vi "pco.camera_LightSheet_Example.vi"() -> ()   [LabVIEW 2020]
uses:
  Camera.lvclass
  SpecialCommandsEdge.lvlib
panel:
  out "colormap(U8)":u32[](array[numeric])
  out "Image(U16)":u16[][](graph)
  in  "Zoom [%]":i32(c297)=26
  out "Image":picture
  in  "dwExposureLines":u32=100
  in  "wTimeBase":u16(ring)=1 items=["ns", "us", "ms"]
  in  "dwLineTime":u32=50
  out "rawImage":u16[][](array[numeric])
  in  "data_format":T1(ring)=enum."Mono16"
  in  "Image Index":u32 max=9
  out "Recorded Images":u32
  in  "Quit":bool
  in  "roiY1":u64=2 min=2 max=2160 step=1
  in  "roiX1":u64=2 min=2 max=2560 step=1
  in  "roiY0":u64=1 min=1 max=2159 step=1
  in  "roiX0":u64=1 min=1 max=2559 step=1
  out "Image Height":u64
  out "Image Width":u64
  in  "dwImgCount":u32=10 caption="Required Number of Images" max=4023
  out "Error":errorcluster {"code" format="%x"}
  # "This example is similar to the simple example, but uses get/set line timeing for controlling the exposure.\nExposureTime = LineTime * ExposureLines\nBeside of the line timing part, a simple recording of an image sequence and the image access afterwards is done.\nIt is a good starting point for writing own applications, especially  for light sheet application development.\nBut it will not be fail save, i.e. doesnt react on errors, just handles them forward to the end\n\nUsage:\nSelect your required image count and the required line tiime + number of exposure lines before you start the program.\nOnce started, the camera class will be initialized and images will be recorded automatically.\nWhen acquisition has finished you can address the images and set a certain roi \nTo finish the program click on quit application, this will force fan exit of the camera class"
  # "pco.labview"
  # "Camera Setup"
  # "Recording Control"
  # "Parameters for image readout"
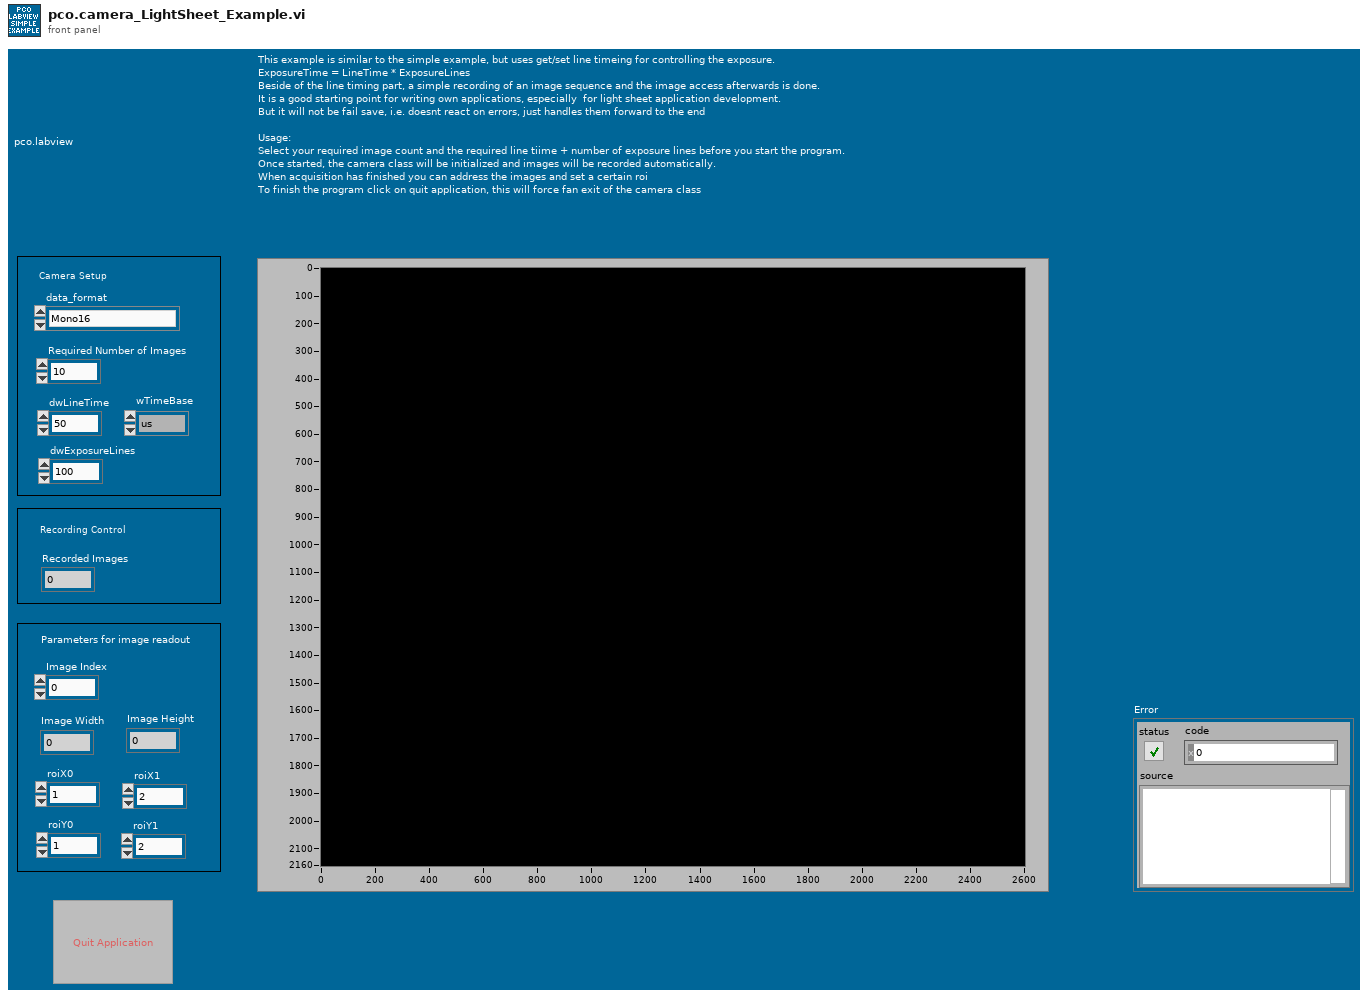
[diagram p1: front panel]
types:
  T1 = enum16{"Undefined", "Mono8", "Mono16", "BGRA8", "RGBA8", "BGRA16", "RGBA16", "CompressedMono8"}
  T2 = enum8{"Enabled", "Disabled", "Disabled and Grayed Out"}
  T3 = enum16{"sequence", "sequence non blocking", "ring buffer", "fifo", "sequence_dpcore", "sequence_non_blocking_dpcore", "ring_buffer_dpcore", "fifo_dpcore", "tif", "multitif", "pcoraw", "b16", "dicom", "multidicom"}
  T4 = typedef "Camera.lvclass/binning.ctl" = cluster{"vert":u16, "horz":u16}
  T5 = cluster{"exposure_time_s":dbl, "delay_time_s":dbl, "roi":cluster{"x0":u64, "y0":u64, "x1":u64, "y1":u64}, "timestamp_mode":u16, "pixelrate":u32, "trigger_mode":u16, "acquire_mode":u16, "metadata_mode":u16, "noisefilter_mode":u16, "binning":T4}
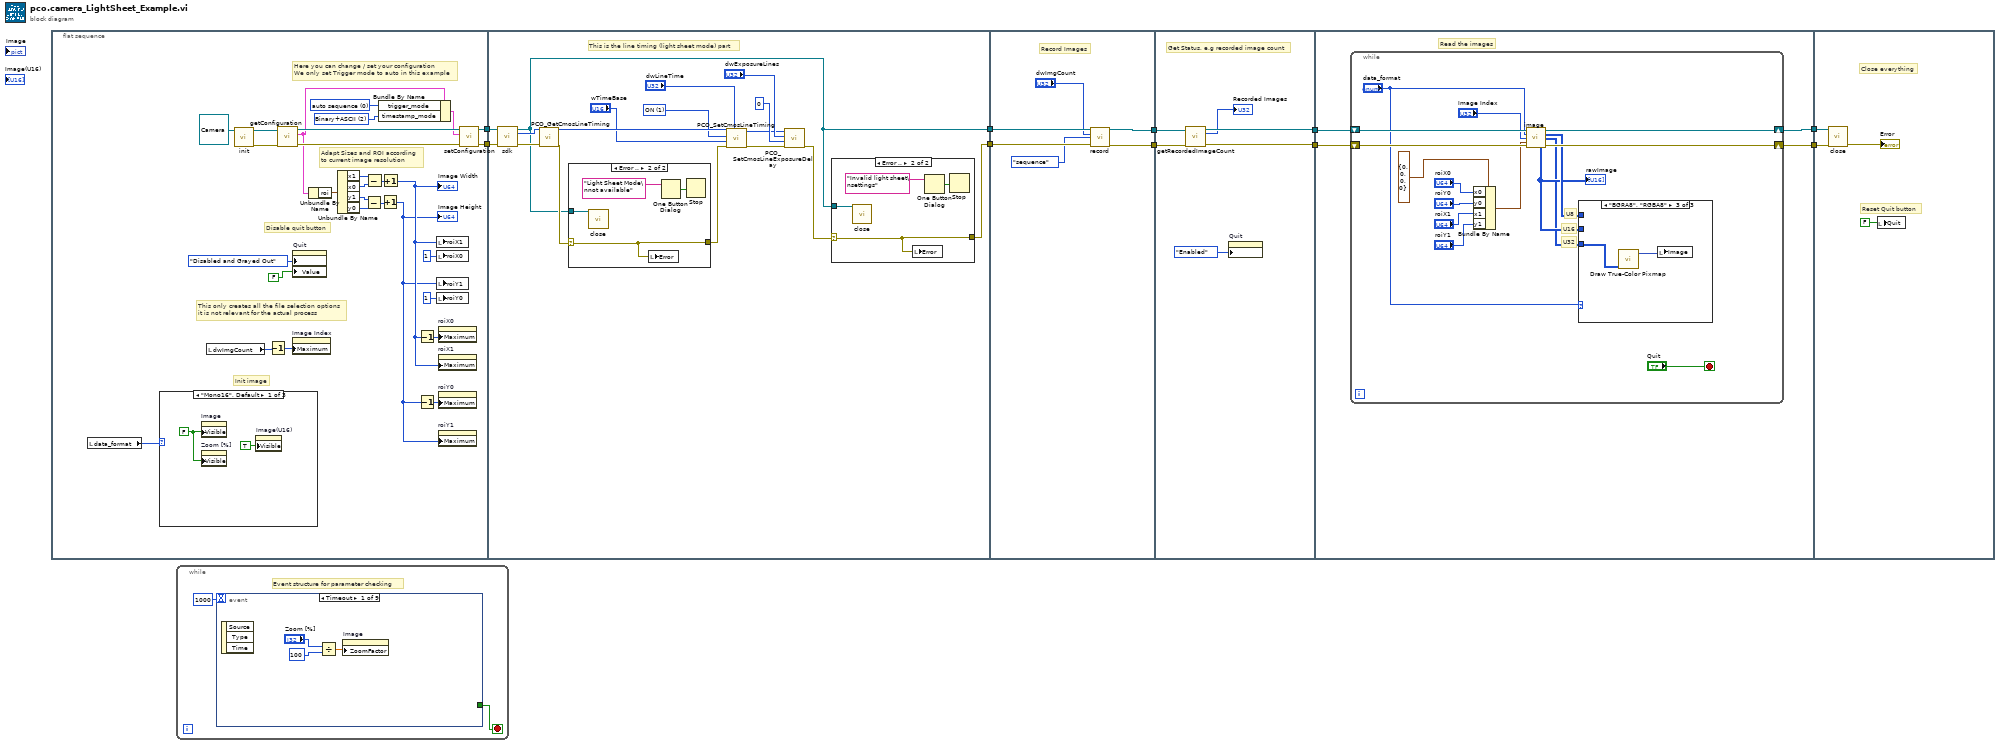
[diagram p0: block diagram]
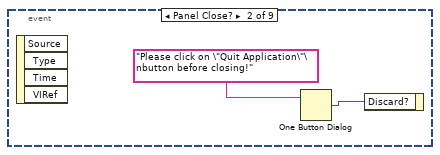
[diagram p2: hidden frame]
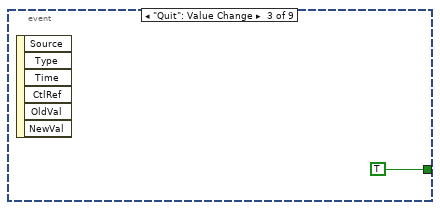
[diagram p3: hidden frame]
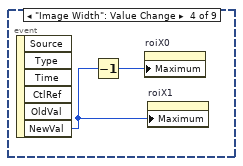
[diagram p4: hidden frame]
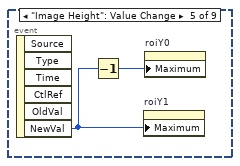
[diagram p5: hidden frame]
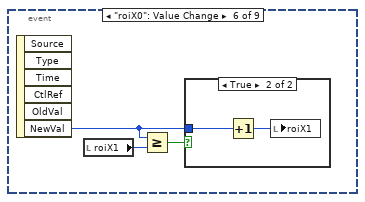
[diagram p6: hidden frame]
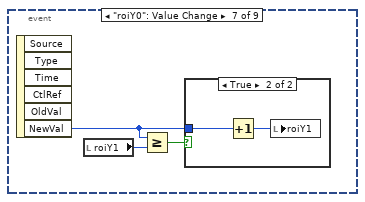
[diagram p8: hidden frame]
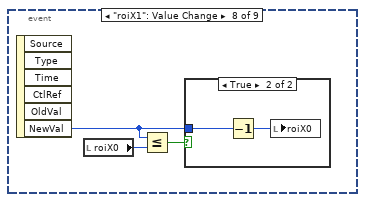
[diagram p10: hidden frame]
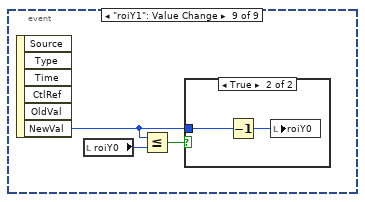
[diagram p12: hidden frame]
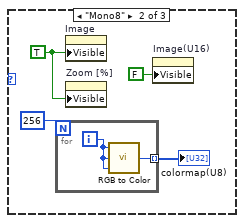
[diagram p14: hidden frame]
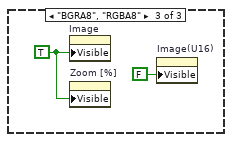
[diagram p15: hidden frame]
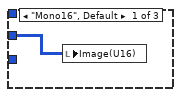
[diagram p18: hidden frame]
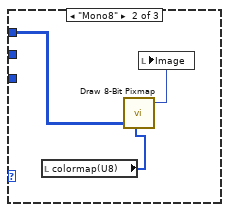
[diagram p19: hidden frame]
diagram:
  n1 = flat-sequence {
    tunnel: [w32] -> w4
    tunnel: [w31] -> w2
    tunnel: w4 -> [w62]
    tunnel: [w52] -> w3
    tunnel: w2 -> [w61]
    tunnel: [w50] -> w1
    tunnel: w3 -> [w82]
    tunnel: w1 -> [w81]
    tunnel: [w79] -> w10
    tunnel: [w78] -> w9
    tunnel: w10 -> [w88]
    tunnel: w9 -> [w87]
    tunnel: [w86] -> w8
    tunnel: [w85] -> w7
    tunnel: w8 -> [w91]
    tunnel: w7 -> [w92]
    tunnel: [w90] -> w6
    tunnel: [w89] -> w5
    tunnel: w6 -> [w116]
    tunnel: w5 -> [w115]
    frame #0 {
      w16 = u16 2 items=["OFF", "Binary", "Binary+ASCII", "ASCII"] ("TimestampMode")
      w36 = u16 0 items=["auto sequence"=0, "software trigger"=1, "external exposure start & software trigger"=2, "external exposure control"=3, "external synchronized"=4, "fast external exposure control"=5, "external CDS control"=6, "slow external exposure control"=7, "external synchronized HDSDI"=258] ("TriggerMode")
      # "Init image"
      # "This only creates all the file selection options\nit is not relevant for the actual process"
      # "Adapt Sizes and ROI according\nto current image resolution"
      # "Disable quit button"
      # "Here you can change / set your configuration\nWe only set Trigger mode to auto in this example"
      n2 = local read "data_format"() -> (w11:T1)
      n3 = case shown="\"Mono16\", Default" w11 {
        frame "Mono16", Default {
          w40 = FALSE ("Visible")
          n4 = property on="Image" class="Pict"("Visible"=w40) -> ()  [unwired: 2 in, 2 out]
          n5 = property on="Zoom [%]" class="Scroll (strict)"("Visible"=w40) -> ()  [unwired: 2 in, 2 out]
          n6 = property on="Image(U16)" class="IntGraph (strict)"("Visible"=TRUE) -> ()  [unwired: 2 in, 2 out]
        }
        frame "Mono8" {
          w44 = TRUE ("Visible")
          n7 = for {
            N: 256 -> [_]
            tunnel: [w46] -> w43 mode=indexing
            i -> [w47]
            n8 = call "RGB to Color.vi"("B"=w47, "G"=w47, "R"=w47) -> ("Color"=w46:u32)
          }
          "colormap(U8)" <- w43
          n9 = property on="Image" class="Pict"("Visible"=w44) -> ()  [unwired: 2 in, 2 out]
          n10 = property on="Zoom [%]" class="Scroll (strict)"("Visible"=w44) -> ()  [unwired: 2 in, 2 out]
          n11 = property on="Image(U16)" class="IntGraph (strict)"("Visible"=FALSE) -> ()  [unwired: 2 in, 2 out]
        }
        frame "BGRA8", "RGBA8" {
          w48 = TRUE ("Visible")
          n12 = property on="Image" class="Pict"("Visible"=w48) -> ()  [unwired: 2 in, 2 out]
          n13 = property on="Zoom [%]" class="Scroll (strict)"("Visible"=w48) -> ()  [unwired: 2 in, 2 out]
          n14 = property on="Image(U16)" class="IntGraph (strict)"("Visible"=FALSE) -> ()  [unwired: 2 in, 2 out]
        }
      }
      n15 = local read "dwImgCount"() -> (w12:u32)
      n16 = call-dynamic "init.vi"("Camera in"=refnum<class "Camera.lvclass"> refnum ("PCOCamera in")) -> ("Camera out"=w38:refnum<class "Camera.lvclass">, "error out"=w37:errorcluster)  [unwired: 8 in]
      n17 = Decrement(x=w12) -> (x-1=w13:u32)
      n18 = call-dynamic "getConfiguration.vi"("error in (no error)"=w37, "Camera in"=w38) -> ("error out"=w34:errorcluster, "configuration"=w26:T5, "Camera out"=w35:refnum<class "Camera.lvclass">)  [unwired: 7 in]
      n19 = property on="Image Index" class="DigNum (strict)"("Maximum"=w13) -> ()  [unwired: 2 in, 2 out]
      n20 = property on="Quit" class="Bool (strict)"("DisabledEnum"=T2."Disabled and Grayed Out" ("Disabled"), "Value"=FALSE ("Stop")) -> ()  [unwired: 2 in, 2 out]
      n21 = Unbundle By Name(w26) -> ("roi"=w25:cluster{"x0":u64, "y0":u64, "x1":u64, "y1":u64})
      n22 = Unbundle By Name(w25) -> ("x1"=w23:u64, "x0"=w24:u64, "y1"=w21:u64, "y0"=w22:u64)
      n23 = Subtract(x=w21, y=w22) -> (x-y=w19:u64)
      n24 = Subtract(x=w23, y=w24) -> (x-y=w20:u64)
      n25 = Bundle By Name(cluster=w26, "trigger_mode"=w36, "timestamp_mode"=w16) -> (w33:T5)
      n26 = Increment(x=w19) -> (x+1=w17:u64)
      "Image Height" <- w17
      n27 = Increment(x=w20) -> (x+1=w18:u64)
      "Image Width" <- w18
      n28 = Decrement(x=w18) -> (x-1=w28:u64)
      n29 = Decrement(x=w17) -> (x-1=w27:u64)
      n30 = local write "roiX1"(w18) -> ()
      n31 = local write "roiX0"(u64 1 ("roiY0")) -> ()
      n32 = local write "roiY1"(w17) -> ()
      n33 = local write "roiY0"(u64 1 ("roiY0")) -> ()
      n34 = property on="roiX0" class="DigNum (strict)"("Maximum"=w28) -> ()  [unwired: 2 in, 2 out]
      n35 = property on="roiX1" class="DigNum (strict)"("Maximum"=w18) -> ()  [unwired: 2 in, 2 out]
      n36 = property on="roiY0" class="DigNum (strict)"("Maximum"=w27) -> ()  [unwired: 2 in, 2 out]
      n37 = property on="roiY1" class="DigNum (strict)"("Maximum"=w17) -> ()  [unwired: 2 in, 2 out]
      n38 = call-dynamic "setConfiguration.vi"("error in (no error)"=w34, "configuration"=w33, "Camera in"=w35) -> ("error out"=w31:errorcluster, "Camera out"=w32:refnum<class "Camera.lvclass">)  [unwired: 7 in]
    }
    frame #1 {
      w58 = u16 1 items=["OFF", "ON"] ("wParameter")
      # "This is the line timing (light sheet mode) part"
      n39 = call-dynamic "sdk.vi"("Camera in"=w62, "error in (no error)"=w61) -> ("Camera out"=w52:refnum<class "Camera.lvclass">, "sdk"=w60:u64, "error out"=w66:errorcluster)  [unwired: 11 in]
      n40 = call "PCO_GetCmosLineTiming.vi"("ph"=w60, "error in (no error)"=w66) -> ("ph out"=w59:u64, "error out"=w65:errorcluster)  [unwired: 10 in, 6 out]
      n41 = case shown="Error .." w65 {
        selector: w65 -> [w72 w73]
        tunnel: [w72 w73] -> w64
        tunnel: w52 -> [_ w74]
        frame No Error {
        }
        frame Error {
          n42 = call-dynamic "close.vi"("Camera in"=w74) -> ()  [unwired: 10 in, 1 out]
          n43 = local write "Error"(w73) -> ()
          n44 = One Button Dialog(message="Light Sheet Mode\nnot available") -> (true=w75:bool)  [unwired: 1 in]
          n45 = Stop(stop? (T)=w75) -> ()
        }
      }
      n46 = call "PCO_SetCmosLineTiming.vi"("dwLineTime"="dwLineTime", "error in (no error)"=w64, "wTimeBase"="wTimeBase", "wParameter"=w58, "ph"=w59) -> ("error out"=w63:errorcluster, "ph out"=w53:u64)  [unwired: 4 in, 1 out]
      n47 = call "PCO_SetCmosLineExposureDelay.vi"("error in (no error)"=w63, "dwDelayLines"=u32 0, "dwExposureLines"="dwExposureLines", "ph"=w53) -> ("error out"=w51:errorcluster)  [unwired: 5 in, 2 out]
      n48 = case shown="Error .." w51 {
        selector: w51 -> [w67 w68]
        tunnel: [w67 w68] -> w50
        tunnel: w52 -> [_ w69]
        frame No Error {
        }
        frame Error {
          n49 = call-dynamic "close.vi"("Camera in"=w69) -> ()  [unwired: 10 in, 1 out]
          n50 = local write "Error"(w68) -> ()
          n51 = One Button Dialog(message="Invalid light sheet\nsettings") -> (true=w70:bool)  [unwired: 1 in]
          n52 = Stop(stop? (T)=w70) -> ()
        }
      }
    }
    frame #2 {
      # "Record Images"
      n53 = call-dynamic "record.vi"("Camera in"=w82, "num_images"="dwImgCount", "record_mode"=T3."sequence", "error in (no error)"=w81) -> ("Camera out"=w79:refnum<class "Camera.lvclass">, "error out"=w78:errorcluster)  [unwired: 10 in]
    }
    frame #3 {
      # "Get Status, e.g recorded image count"
      n54 = call-dynamic "getRecordedImageCount.vi"("Camera in"=w88, "error in (no error)"=w87) -> ("Camera out"=w86:refnum<class "Camera.lvclass">, "recorded_image_count"=→"Recorded Images":u32, "error out"=w85:errorcluster)  [unwired: 11 in]
      n55 = property on="Quit" class="Bool (strict)"("DisabledEnum"=T2."Enabled" ("Disabled")) -> ()  [unwired: 2 in, 2 out]
    }
    frame #4 {
      # "Read the images"
      n56 = while {
        shift-right: [w106] -> w90
        shift-left: w91 -> [w108]
        shift-right: [w101] -> w89
        shift-left: w92 -> [w107]
        stop <- "Quit" stop-if-true
        # "U32"
        # "U16"
        # "U8"
        n57 = Bundle By Name(cluster=cluster{"x0":u64, "y0":u64, "x1":u64, "y1":u64} {"x0"=0, "y0"=0, "x1"=0, "y1"=0} ("roi"), "x0"="roiX0", "y0"="roiY0", "x1"="roiX1", "y1"="roiY1") -> (w100:cluster{"x0":u64, "y0":u64, "x1":u64, "y1":u64})
        n58 = call-dynamic "image.vi"("Camera in"=w108, "data_format"="data_format", "image_index"="Image Index", "roi"=w100, "error in (no error)"=w107) -> ("Camera out"=w106:refnum<class "Camera.lvclass">, "image (U8)"=w97:u8[][], "image (U32)"=w95:u32[][], "raw_image (U16)"=w96:u16[][], "error out"=w101:errorcluster)  [unwired: 3 in, 3 out]
        "rawImage" <- w96
        n59 = case shown="\"BGRA8\", \"RGBA8\"" "data_format" {
          tunnel: w95 -> [_ _ w114]
          tunnel: w97 -> [_ w110 _]
          tunnel: w96 -> [w109 _ _]
          frame "Mono16", Default {
            n60 = local write "Image(U16)"(w109) -> ()
          }
          frame "Mono8" {
            n61 = local read "colormap(U8)"() -> (w112:u32[])
            n62 = call "Draw 8-Bit Pixmap.vi"("data"=w110, "color table"=w112) -> ("new picture"=w111:picture)  [unwired: 7 in]
            n63 = local write "Image"(w111) -> ()
          }
          frame "BGRA8", "RGBA8" {
            n64 = call "Draw True-Color Pixmap.vi"("data (RGB format)"=w114) -> ("new picture"=w113:picture)  [unwired: 8 in]
            n65 = local write "Image"(w113) -> ()
          }
        }
      }
    }
    frame #5 {
      # "Reset Quit button"
      # "Close everything"
      n66 = call-dynamic "close.vi"("error in (no error)"=w115, "Camera in"=w116) -> ("error out"=→"Error":errorcluster)  [unwired: 9 in]
      n67 = local write "Quit"(FALSE ("Stop")) -> ()
    }
  }
  n68 = while {
    stop <- w119 stop-if-true
    # "Event structure for parameter checking"
    n69 = event shown="[0] Timeout" {
      selector: _ -> [_ _ _ _ _ _ _ _ _]
      dyn-events: _ -> [_ _ _ _ _ _ _ _ _]
      timeout: 1000 -> [_ _ _ _ _ _ _ _ _]
      tunnel: [_ _ TRUE _ _ _ _ _ _] -> w119
      event Timeout {
        n70 = event-data() -> ()  [unwired: 1 in, 3 out]
        n71 = Divide(x="Zoom [%]", y=100 ("Zoom [%]")) -> (x/y=w122:dbl)
        n72 = property on="Image" class="Pict"("ZoomFactor"=w122) -> ()  [unwired: 2 in, 2 out]
      }
      event Panel Close? {
        n73 = event-data() -> ()  [unwired: 1 in, 4 out]
        n74 = One Button Dialog(message="Please click on \"Quit Application\"\nbutton before closing!") -> (true=w124:bool)  [unwired: 1 in]
        n75 = event-data("Discard?"=w124) -> ()  [unwired: 1 in, 1 out]
      }
      event "Quit": Value Change {
        n76 = event-data() -> ()  [unwired: 1 in, 6 out]
      }
      event "Image Width": Value Change {
        n77 = event-data() -> ("NewVal"=w127:u64)  [unwired: 1 in, 5 out]
        n78 = Decrement(x=w127) -> (x-1=w128:u64)
        n79 = property on="roiX0" class="DigNum (strict)"("Maximum"=w128) -> ()  [unwired: 2 in, 2 out]
        n80 = property on="roiX1" class="DigNum (strict)"("Maximum"=w127) -> ()  [unwired: 2 in, 2 out]
      }
      event "Image Height": Value Change {
        n81 = event-data() -> ("NewVal"=w129:u64)  [unwired: 1 in, 5 out]
        n82 = Decrement(x=w129) -> (x-1=w130:u64)
        n83 = property on="roiY1" class="DigNum (strict)"("Maximum"=w129) -> ()  [unwired: 2 in, 2 out]
        n84 = property on="roiY0" class="DigNum (strict)"("Maximum"=w130) -> ()  [unwired: 2 in, 2 out]
      }
      event "roiX0": Value Change {
        n85 = event-data() -> ("NewVal"=w131:u64)  [unwired: 1 in, 5 out]
        n86 = local read "roiX1"() -> (w133:u64)
        n87 = Greater Or Equal?(x=w131, y=w133) -> (x >= y?=w132:bool)
        n88 = case shown="True" w132 {
          tunnel: w131 -> [_ w135]
          frame False {
          }
          frame True {
            n89 = Increment(x=w135) -> (x+1=w134:u64)
            n90 = local write "roiX1"(w134) -> ()
          }
        }
      }
      event "roiY0": Value Change {
        n91 = event-data() -> ("NewVal"=w136:u64)  [unwired: 1 in, 5 out]
        n92 = local read "roiY1"() -> (w138:u64)
        n93 = Greater Or Equal?(x=w136, y=w138) -> (x >= y?=w137:bool)
        n94 = case shown="True" w137 {
          tunnel: w136 -> [_ w140]
          frame False {
          }
          frame True {
            n95 = Increment(x=w140) -> (x+1=w139:u64)
            n96 = local write "roiY1"(w139) -> ()
          }
        }
      }
      event "roiX1": Value Change {
        n97 = event-data() -> ("NewVal"=w141:u64)  [unwired: 1 in, 5 out]
        n98 = local read "roiX0"() -> (w143:u64)
        n99 = Less Or Equal?(x=w141, y=w143) -> (x <= y?=w142:bool)
        n100 = case shown="True" w142 {
          tunnel: w141 -> [_ w145]
          frame False {
          }
          frame True {
            n101 = Decrement(x=w145) -> (x-1=w144:u64)
            n102 = local write "roiX0"(w144) -> ()
          }
        }
      }
      event "roiY1": Value Change {
        n103 = event-data() -> ("NewVal"=w146:u64)  [unwired: 1 in, 5 out]
        n104 = local read "roiY0"() -> (w148:u64)
        n105 = Less Or Equal?(x=w146, y=w148) -> (x <= y?=w147:bool)
        n106 = case shown="True" w147 {
          tunnel: w146 -> [_ w150]
          frame False {
          }
          frame True {
            n107 = Decrement(x=w150) -> (x-1=w149:u64)
            n108 = local write "roiY0"(w149) -> ()
          }
        }
      }
    }
  }
